vi "CYLL(SubVI).vi"(1 "N cycles":dbl, 2 "Cycling\ntemperature":u16) -> (0 "cycle life losses(%)":dbl)   [LabVIEW 2017]
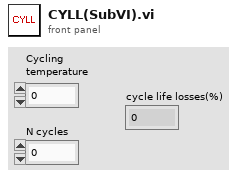
[diagram p1: front panel]
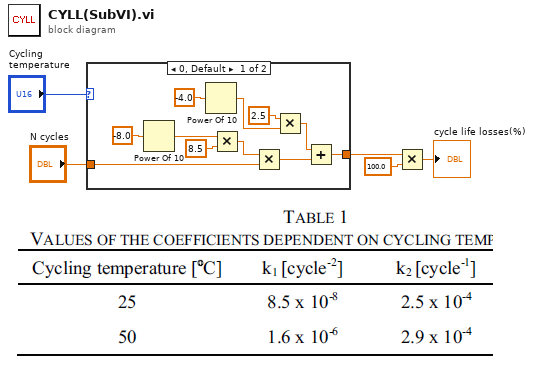
[diagram p0: block diagram]
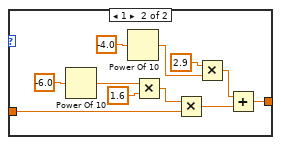
[diagram p2: hidden frame]
diagram:
  n1 = case shown="0, Default" "Cycling\ntemperature" {
    tunnel: [w6 w18] -> w2
    tunnel: "N cycles" -> [w7 w17]
    frame 0, Default {
      n2 = Power Of 10(x=-8.0) -> (10^x=w11:dbl)
      n3 = Power Of 10(x=-4.0) -> (10^x=w10:dbl)
      n4 = Multiply(x=w11, y=8.5) -> (x*y=w13:dbl)
      n5 = Multiply(x=w13, y=w7) -> (x*y=w16:dbl)
      n6 = Multiply(x=2.5, y=w10) -> (x*y=w8:dbl)
      n7 = Add(x=w8, y=w16) -> (x+y=w6:dbl)
    }
    frame 1 {
      n8 = Power Of 10(x=-6.0) -> (10^x=w22:dbl)
      n9 = Power Of 10(x=-4.0) -> (10^x=w21:dbl)
      n10 = Multiply(x=w22, y=1.6) -> (x*y=w24:dbl)
      n11 = Multiply(x=w24, y=w17) -> (x*y=w27:dbl)
      n12 = Multiply(x=2.9, y=w21) -> (x*y=w19:dbl)
      n13 = Add(x=w19, y=w27) -> (x+y=w18:dbl)
    }
  }
  n14 = Multiply(x=w2, y=100.0) -> (x*y=→"cycle life losses(%)":dbl)
